vi "QWavelength.vi"(8 "error in (no error)":errorcluster, 11 "VISA resource name":refnum<visa-resource-name>) -> (0 "error out":errorcluster, 2 "Wavelength":dbl[unit], 3 "VISA resource name out":refnum<visa-resource-name>)   [LabVIEW 2009, in "Newport 1830-C.lvlib"]
doc: "Returns current wavelength setting"
uses:
  Newport 1830-C.lvlib
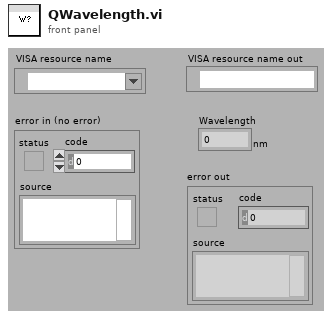
[diagram p1: front panel]
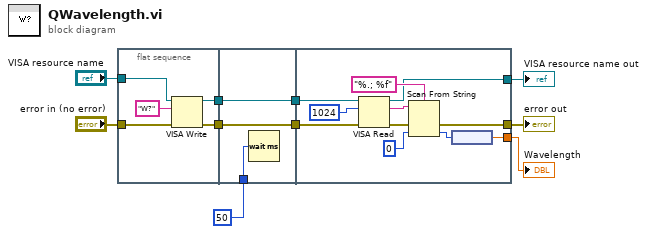
[diagram p0: block diagram]
diagram:
  n1 = flat-sequence {
    tunnel: [w14] -> w6
    tunnel: [w13] -> w5
    tunnel: "VISA resource name" -> [w12]
    tunnel: "error in (no error)" -> [w11]
    tunnel: [w18] -> w7
    tunnel: w6 -> [w18]
    tunnel: w5 -> [w17]
    tunnel: [w17] -> w4
    tunnel: u32 50 ("Delay Time (s)") -> [w16]
    tunnel: [w23] -> w10
    tunnel: [w22] -> w9
    tunnel: [w21] -> w8
    tunnel: w7 -> [w20]
    tunnel: w4 -> [w19]
    frame #0 {
      n2 = VISA Write(VISA resource name=w12, write buffer="W?" ("command"), error in (no error)=w11) -> (VISA resource name out=w14:refnum<visa-resource-name>, error out=w13:errorcluster)  [unwired: 1 out]
    }
    frame #1 {
      n3 = Wait (ms)(milliseconds to wait=w16) -> ()  [unwired: 1 out]
    }
    frame #2 {
      n4 = VISA Read(VISA resource name=w20, byte count=u32 1024, error in (no error)=w19) -> (VISA resource name out=w23:refnum<visa-resource-name>, read buffer=w25:string, error out=w27:errorcluster)  [unwired: 1 out]
      n5 = Scan From String(format string="%.; %f", input string=w25, error in=w27, default 1=0 ("default value 1")) -> (error out=w22:errorcluster, output 1=w29:i32)  [unwired: 1 in, 2 out]
      n6 = node(w29) -> (w21:dbl[unit])
    }
  }
  "Wavelength" <- w8
  "error out" <- w9
  "VISA resource name out" <- w10
